vi "Compute.vi"(8 "error in (no error)":errorcluster, 9 "Data Channels":T1, 10 "x-var":dbl, 11 "Normalize in":refnum<class "Normalize.lvclass">) -> (0 "error out":errorcluster, 1 "Add'l Data Channels":T1, 3 "Normalize out":refnum<class "Normalize.lvclass">)   [LabVIEW 2009, in "Normalize.lvclass"]
doc: "Given a data channel and an x-coordinate, compute and return one or more new data channels."
uses:
  Normalize.lvclass
  Instruments/Utility Classes/Readable/Data Channels.ctl
  Instruments/Utility Classes/Readable/Data Channel.ctl
  Instruments/Utility Classes/Readable/Data Point.ctl
  Aux Data Source/Aux Data Source.lvclass
  Instruments/Utility Classes/Readable/Readable.lvclass
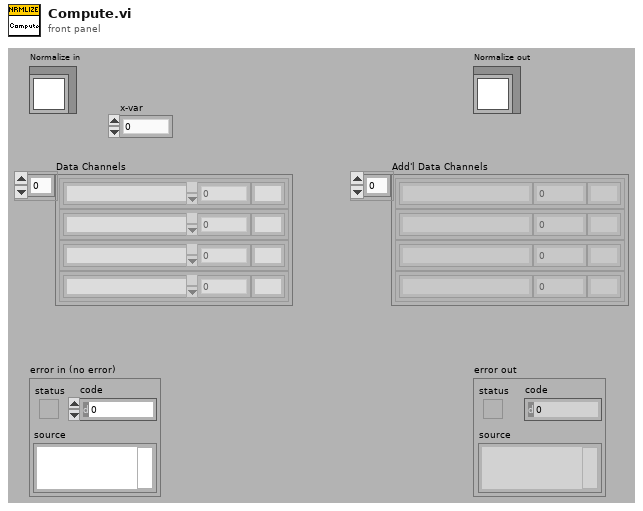
[diagram p1: front panel]
types:
  T1 = typedef "Readable.lvclass/Data Channels.ctl" = T2[]
  T2 = typedef "Readable.lvclass/Data Channel.ctl" = cluster{"Name":string, "Data Point":T3, "Unit":string}
  T3 = typedef "Readable.lvclass/Data Point.ctl" = dbl
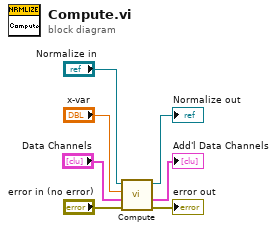
[diagram p0: block diagram]
diagram:
  n1 = call-parent "Compute.vi"("error in (no error)"="error in (no error)", "Data Channels"="Data Channels", "x-var"="x-var", "Aux Data Source in"="Normalize in") -> ("error out"=→"error out":errorcluster, "Add'l Data Channels"=→"Add'l Data Channels":T1, "Aux Data Source out"=→"Normalize out":refnum<class "Normalize.lvclass">)  [unwired: 5 in]
